vi "Cycle Through Images test.vi"() -> ()   [LabVIEW 2020]
panel:
  out "number":i32
  in  "stop number":bool
  out "iterations":i32
  in  "CATCH":bool
  in  "stop catch":bool
  out "number caught":i32
  in  "Image Type":u16(ring) items=["Grayscale (U8)"=0, "Grayscale (I16)"=1, "Grayscale (U16)"=7, "RGB Color (U32)"=4]
  in  "File Path 2":path
  in  "Y Start Position 2":i32
  in  "X Start Position 2":i32
  out "Image":i32
  in  "Next":bool
  out "?":picture
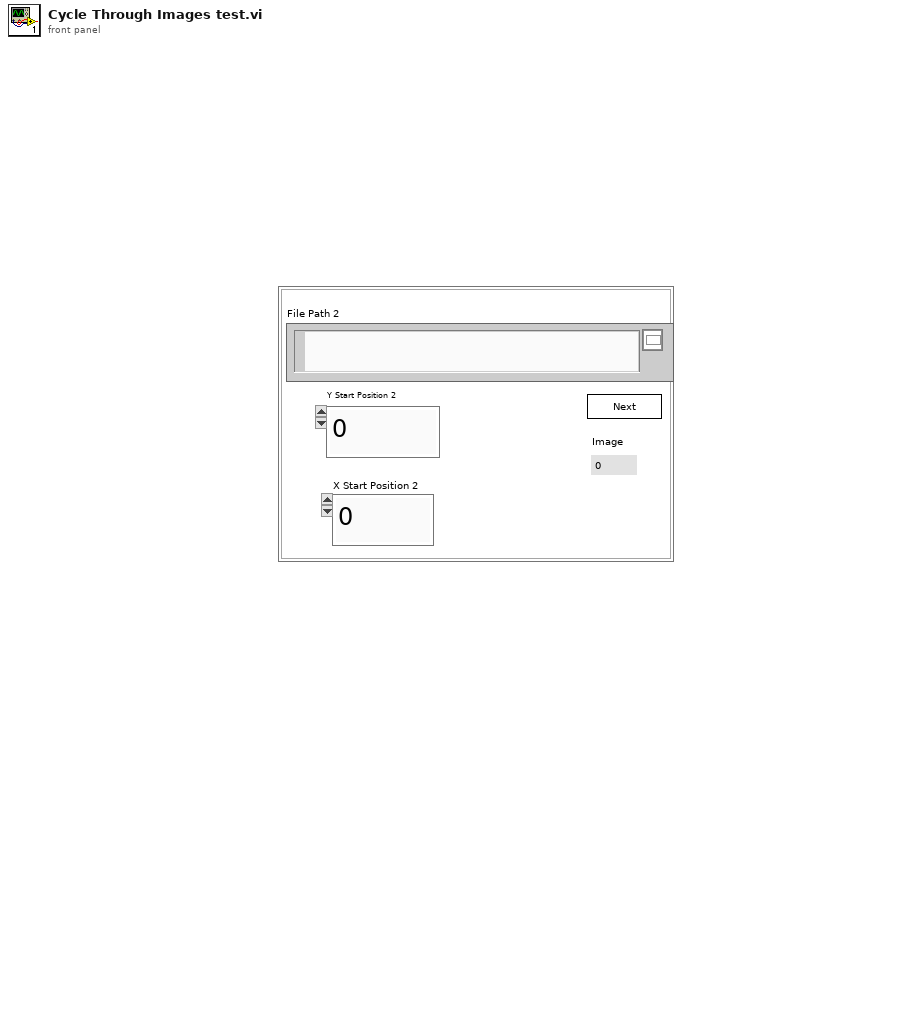
[diagram p1: front panel]
types:
  T1 = typedef "IMAQ Image.ctl" = refnum<image>
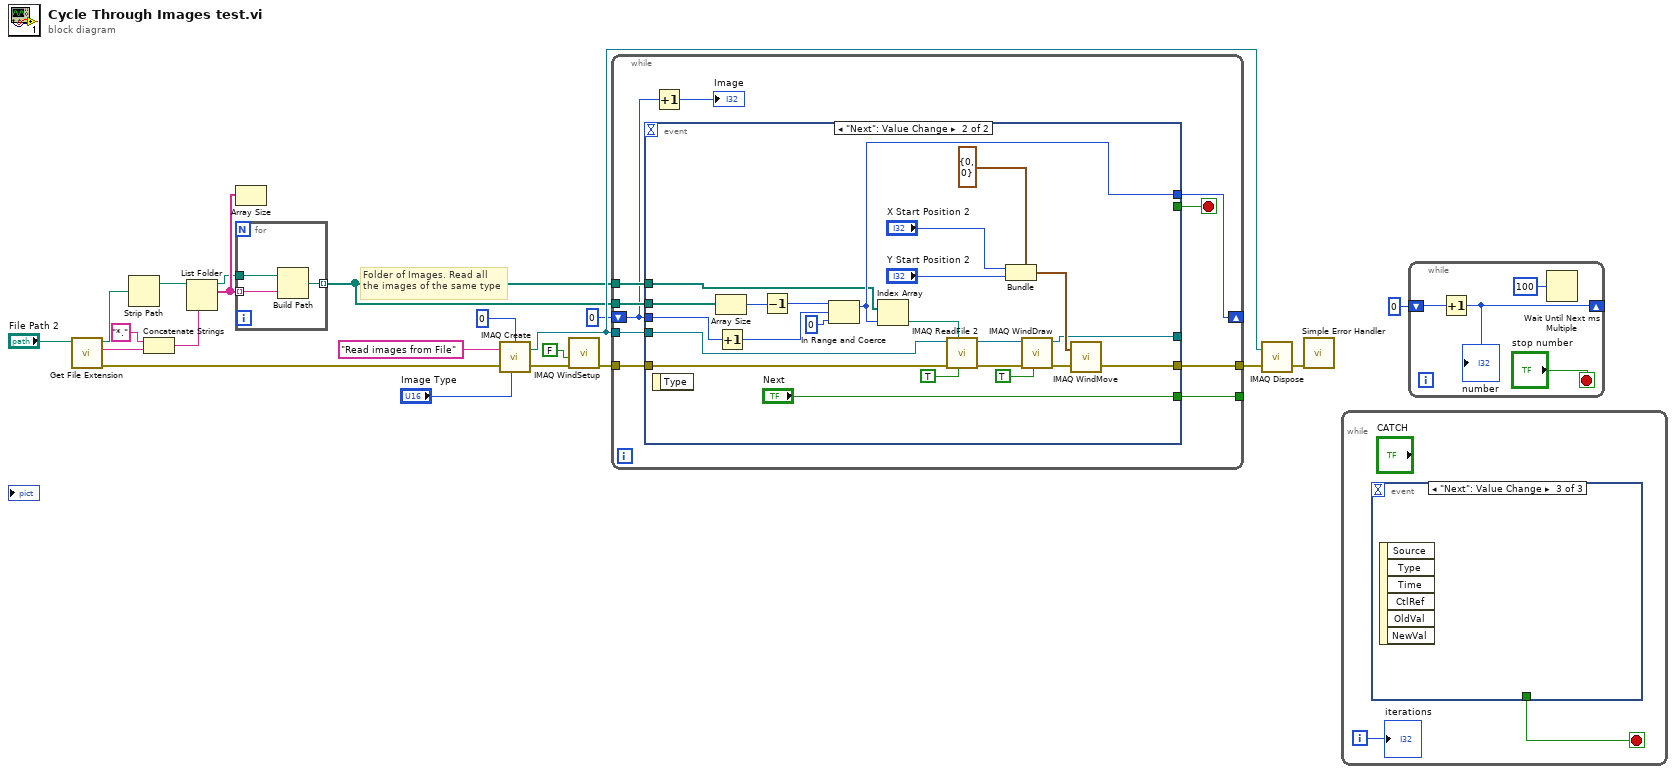
[diagram p0: block diagram]
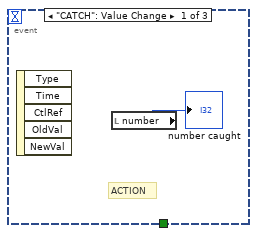
[diagram p2: hidden frame]
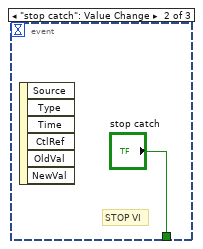
[diagram p3: hidden frame]
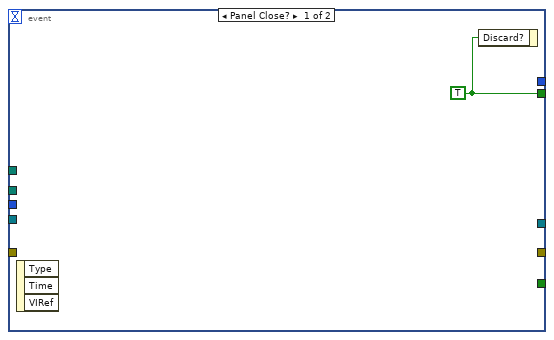
[diagram p4: hidden frame]
diagram:
  # "Folder of Images. Read all the images of the same type"
  n1 = call <vilib>:"Get File Extension.vi"("file"="File Path 2") -> ("error out"=w17:errorcluster, "lowercase file extension"=w15:string, "dup file"=w16:path)  [unwired: 6 in, 2 out]
  n2 = Strip Path(path=w16) -> (stripped path=w9:path)  [unwired: 1 out]
  n3 = Concatenate Strings("*." ("string"), w15) -> (w8:string)
  n4 = List Folder(path=w9, pattern=w8) -> (path out=w6:path, filenames=w7:string[])  [unwired: 2 in, 2 out]
  n5 = Array Size(array=w7) -> ()  [unwired: 1 out]
  n6 = for {
    tunnel: w6 -> [w24]
    tunnel: w7 -> [w23] mode=indexing
    tunnel: [w22] -> w4 mode=indexing
    n7 = Build Path(base path=w24, name or relative path=w23) -> (appended path=w22:path)
  }
  n8 = call "IMAQ Create"("Border Size"=0, "Image Name"="Read images from File", "Image Type"="Image Type", "error in (no error)"=w17) -> ("New Image"=w13:T1, "error out"=w14:errorcluster)  [unwired: 1 in]
  n9 = call "IMAQ WindSetup"("error in (no error)"=w14, "Window has title bar? (Yes)"=FALSE) -> ("error out"=w3:errorcluster)  [unwired: 9 in]
  n10 = while {
    tunnel: w4 -> [w33]
    shift-right: [w32] -> _
    shift-left: 0 -> [w30]
    tunnel: w4 -> [w31]
    tunnel: [w28] -> w20
    tunnel: w3 -> [w27]
    tunnel: w13 -> [w26]
    tunnel: [w25] -> _
    stop <- w34 stop-if-true
    n11 = event shown="[1] \"Next\": Value Change" {
      selector: _ -> [_ _]
      dyn-events: _ -> [_ _]
      timeout: _ -> [_ _]
      tunnel: [w35 _] -> w34
      tunnel: w33 -> [_ w43]
      tunnel: w30 -> [_ w58]
      tunnel: [_ w44] -> w32
      tunnel: w31 -> [_ w55]
      tunnel: [_ w42] -> w28
      tunnel: [_ w41] -> _
      tunnel: w27 -> [_ w40]
      tunnel: w26 -> [_ w39]
      tunnel: [_ "Next"] -> w25
      event Panel Close? {
        w35 = TRUE ("Discard?")
        n12 = event-data() -> ()  [unwired: 1 in, 3 out]
        n13 = event-data("Discard?"=w35) -> ()  [unwired: 1 in, 1 out]
      }
      event "Next": Value Change {
        n14 = event-data() -> ()  [unwired: 1 in, 1 out]
        n15 = Array Size(array=w55) -> (size(s)=w54:i32)
        n16 = Increment(x=w58) -> (x+1=w57:i32)
        n17 = Decrement(x=w54) -> (x-1=w53:i32)
        n18 = In Range and Coerce(upper limit=w53, x=w57, lower limit=0) -> (coerced(x)=w44:i32)  [unwired: 1 out]
        n19 = Index Array(array=w43, index=w44) -> (element=w48:path)
        n20 = call "IMAQ ReadFile 2"("Use File Path Image Type"=TRUE, "File Path"=w48, "error in (no error)"=w40, "Image"=w39) -> ("error out"=w50:errorcluster, "Image Out"=w49:T1)  [unwired: 3 in, 3 out]
        n21 = Bundle(cluster=cluster{"X Position":i32, "Y Position":i32} {"X Position"=0, "Y Position"=0} ("output cluster"), "X Position"="X Start Position 2", "Y Position"="Y Start Position 2") -> (w52:cluster{"X Position":i32, "Y Position":i32})
        n22 = call "IMAQ WindDraw"("Resize to Image Size? (Y)"=TRUE ("Use File Path Image Type"), "error in (no error)"=w50, "Image"=w49) -> ("error out"=w51:errorcluster, "Image Out (duplicate)"=w41:T1)  [unwired: 7 in]
        n23 = call "IMAQ WindMove"("Coordinates (screen)"=w52, "error in (no error)"=w51) -> ("error out"=w42:errorcluster)  [unwired: 3 in, 1 out]
      }
    }
    n24 = Increment(x=w30) -> (x+1=→"Image":i32)
  }
  n25 = call "IMAQ Dispose"("Image"=w13, "error in (no error)"=w20) -> ("error out"=w21:errorcluster)  [unwired: 4 in]
  n26 = call <vilib>:"Simple Error Handler.vi"("error in (no error)"=w21) -> ()  [unwired: 4 in, 5 out]
  n27 = while {
    i -> [w60]
    stop <- w59 stop-if-true
    n28 = event shown="[2] \"Next\": Value Change" {
      selector: _ -> [_ _ _]
      dyn-events: _ -> [_ _ _]
      timeout: _ -> [_ _ _]
      tunnel: [_ "stop catch" _] -> w59
      event "CATCH": Value Change {
        # "ACTION"
        n29 = event-data() -> ()  [unwired: 1 in, 5 out]
        n30 = local read "number"() -> (→"number caught":i32)
      }
      event "stop catch": Value Change {
        # "STOP VI"
        n31 = event-data() -> ()  [unwired: 1 in, 6 out]
      }
      event "Next": Value Change {
        n32 = event-data() -> ()  [unwired: 1 in, 6 out]
      }
    }
    "iterations" <- w60
  }
  n33 = while {
    shift-right: [w65] -> _
    shift-left: 0 -> [w66]
    stop <- "stop number" stop-if-true
    n34 = Increment(x=w66) -> (x+1=w65:i32)
    "number" <- w65
    n35 = Wait Until Next ms Multiple(millisecond multiple=u32 100) -> ()  [unwired: 1 out]
  }
